vi "Parse String.vi"(0 "Ack package":string) -> (2 "Page ID":u16, 4 "Ackmnt":string, 13 "Cmd Suceed?":bool, 14 "Confirmation Code":string)   [LabVIEW 2020]
panel:
  out "Match Score":u16
  out "(hi.lo)":u16
  out "Array":u8[](array[numeric]) format="%.0x"
  out "Confirmation ByteCode":u8 format="%.0x"
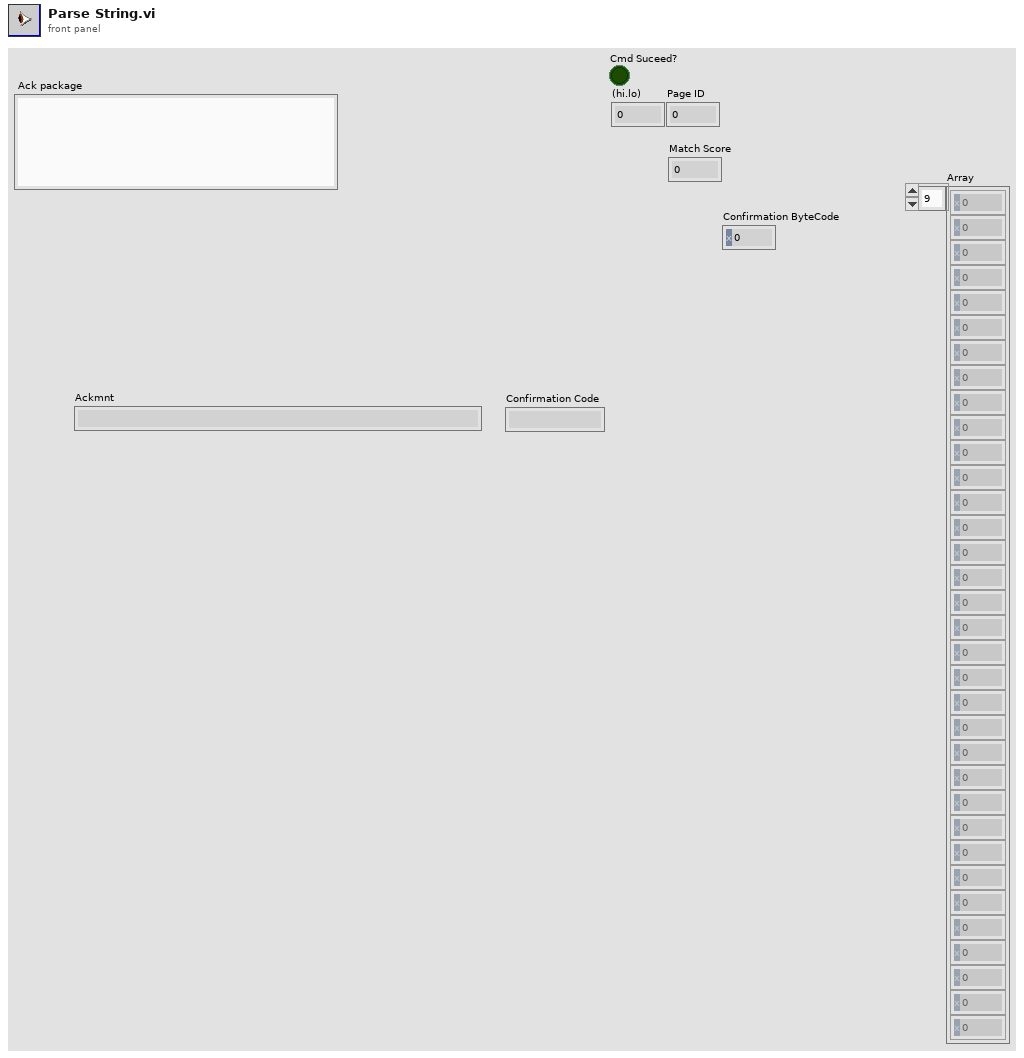
[diagram p1: front panel]
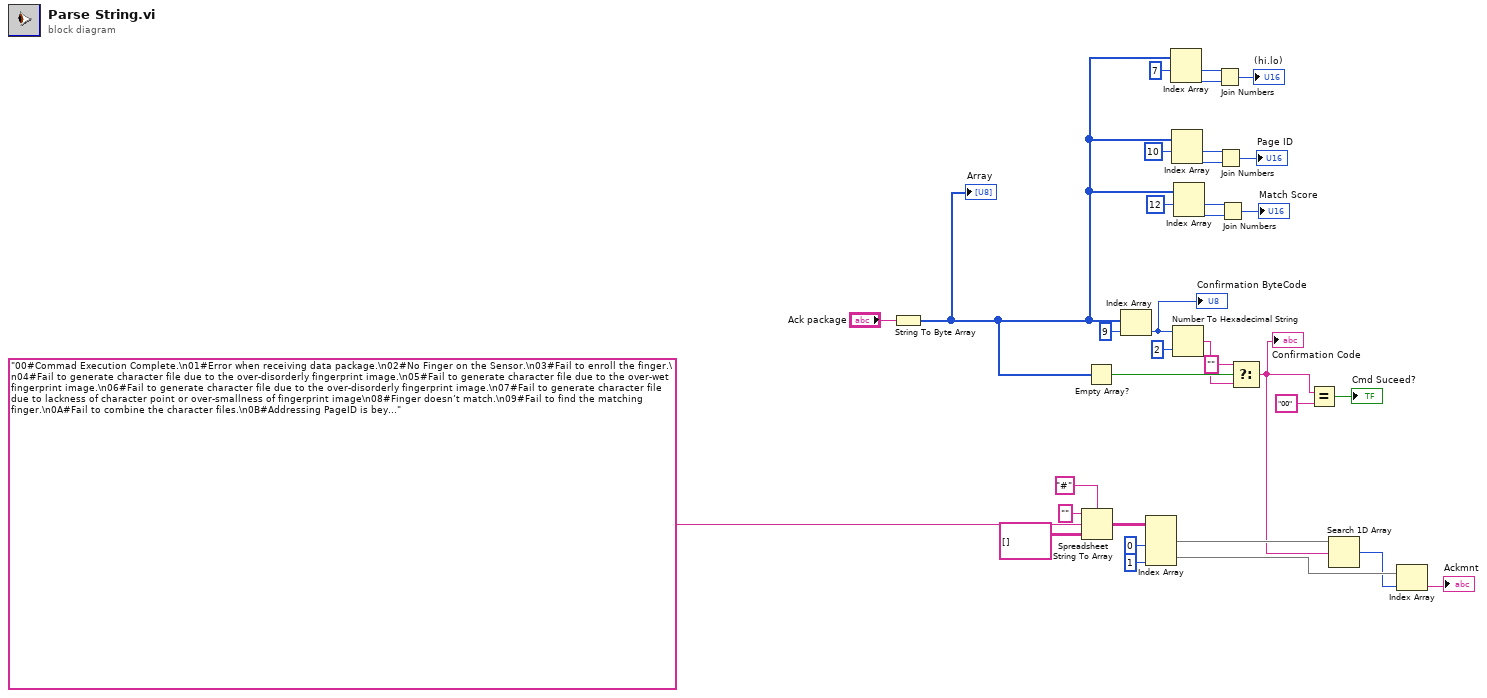
[diagram p0: block diagram]
diagram:
  n1 = String To Byte Array(string="Ack package") -> (unsigned byte array=w5:u8[])
  "Array" <- w5
  n2 = Spreadsheet String To Array(delimiter (Tab)="#", format string="", spreadsheet string="00#Commad Execution Complete.\n01#Error when receiving data package.\n02#No Finger on the Sensor.\n03#Fail to enroll the finger.\n04#Fail to generate character file due to the over-disorderly fingerprint image.\n05#Fail to generate character file due to the over-wet fingerprint image.\n06#Fail to generate character file due to the over-disorderly fingerprint image.\n07#Fail to generate character file due to lackness of character point or over-smallness of fingerprint image\n08#Finger doesn’t match.\n09#Fail to find the matching finger.\n0A#Fail to combine the character files.\n0B#Addressing PageID is beyond the finger library.\n0C#Error when reading template from library or the template is invalid.\n0D#Error when uploading template.\n0E#Module can’t receive the following data packages.\n0F#Error when uploading image.\n10#Fail to delete the template.\n11#Fail to clear finger library.\n13#Wrong password!\n15#Fail to generate the image for the lackness of valid primary image.\n18#Error when writing flash.\n19#No definition error.\n1A#Invalid register number.\n1B#Incorrect configuration of register.\n1C#Wrong notepad page number.\n1D#Fail to operate the communication port.others: system reserved.\n41#No finger on sensor when add fingerprint on second time.\n42#Fail to enroll the finger for second fingerprint add.\n43#Fail to generate character file due to lackness of character point or over-smallness of fingerprint image for second fingerprint add\n44#Fail to generate character file due to the over-disorderly fingerprint image for second fingerprint add.\n45#Duplicate fingerprint", array type (2D Dbl)=string[][] [] ("Array of Strings")) -> (array=w25:string[][])
  n3 = Empty Array?(array=w5) -> (empty?=w4:bool)
  n4 = Index Array(array=w5, index=9) -> (element=w26:u8)
  "Confirmation ByteCode" <- w26
  n5 = Index Array(array=w25, index (col) #1=0 ("disabled index (col)"), index (col) #2=1 ("index (col)")) -> (element #1=w27:string[], element #2=w23:string[])  [unwired: 2 in]
  n6 = Index Array(array=w5, index #1=7 ("index")) -> (element #1=w16:u8, element #2=w15:u8)  [unwired: 1 in]
  n7 = Index Array(array=w5, index #1=10 ("index")) -> (element #1=w12:u8, element #2=w13:u8)  [unwired: 1 in]
  n8 = Number To Hexadecimal String(1:i16 2 ("width (-)"), 2:w26) -> (0:w3:string)
  n9 = Index Array(array=w5, index #1=12 ("index")) -> (element #1=w7:u8, element #2=w6:u8)  [unwired: 1 in]
  n10 = Join Numbers(hi=w16, lo=w15) -> ((hi.lo)=→"(hi.lo)":u16)
  n11 = Join Numbers(hi=w12, lo=w13) -> ((hi.lo)=→"Page ID":u16)
  n12 = Join Numbers(hi=w7, lo=w6) -> ((hi.lo)=→"Match Score":u16)
  n13 = Select(t="", s=w4, f=w3) -> (s? t:f=w1:string)
  "Confirmation Code" <- w1
  n14 = Equal?(x=w1, y="00") -> (x = y?=→"Cmd Suceed?":bool)
  n15 = Search 1D Array(1D array=w27, element=w1) -> (index of element=w22:i32)  [unwired: 1 in]
  n16 = Index Array(array=w23, index=w22) -> (element=→"Ackmnt":string)
